vi "SLM Ctrl Make Plot Data.vi"(7 "Mode Array":dbl[](array[numeric])) -> (4 "Plot Data":cluster{dbl[], dbl[]}, 8 "Min Value":dbl, 15 "Max Value":dbl)   [LabVIEW 2018]
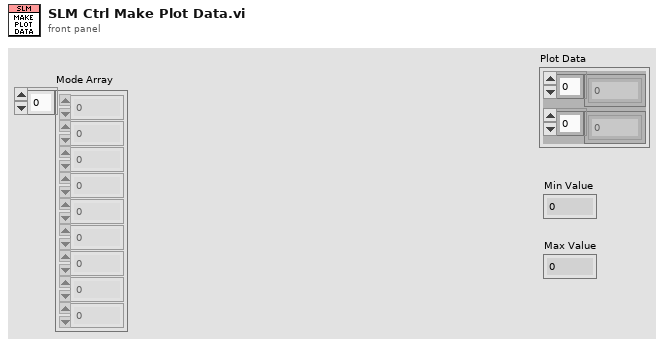
[diagram p1: front panel]
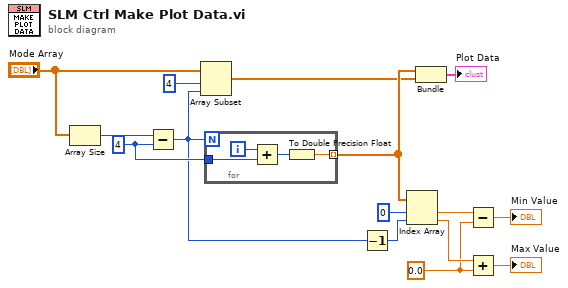
[diagram p0: block diagram]
diagram:
  w2 = 0.0
  w12 = 4 ("y")
  n1 = Array Size(array="Mode Array") -> (size(s)=w13:i32)
  n2 = Subtract(x=w13, y=w12) -> (x-y=w10:i32)
  n3 = Array Subset(array="Mode Array", index=4, length=w10) -> (w7:dbl[])
  n4 = for {
    N: w10 -> [_]
    tunnel: w12 -> [w18]
    tunnel: [w16] -> w8 mode=indexing
    i -> [w19]
    n5 = Add(x=w19, y=w18) -> (x+y=w17:i32)
    n6 = To Double Precision Float(number=w17) -> (double precision float=w16:dbl)
  }
  n7 = Decrement(x=w10) -> (x-1=w9:i32)
  n8 = Index Array(array=w8, index #1=0 ("index"), index #2=w9) -> (element #1=w6:dbl, element #2=w4:dbl)
  n9 = Bundle(w8, w7) -> (→"Plot Data":cluster{dbl[], dbl[]})  [unwired: 1 in]
  n10 = Subtract(x=w6, y=w2) -> (x-y=→"Min Value":dbl)
  n11 = Add(x=w4, y=w2) -> (x+y=→"Max Value":dbl)
